vi "RawToRH.vi"(2 "Data":u8[](array[numeric]), 5 "error in (no error)":errorcluster) -> (16 "RH":dbl, 19 "error out":errorcluster)   [LabVIEW 2019, in "SHT21.lvclass"]
uses:
  SHT21.lvclass
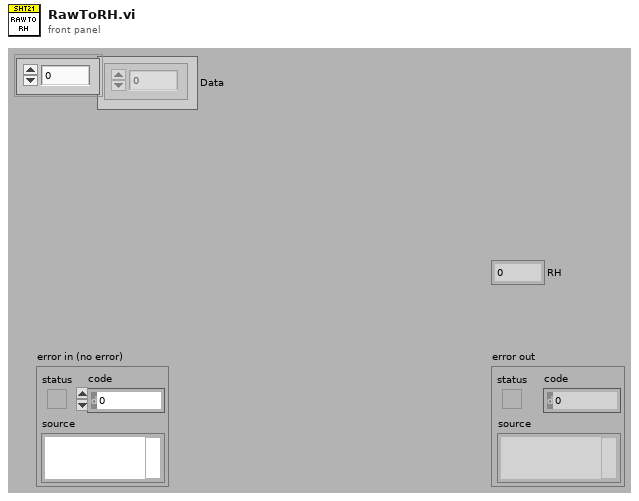
[diagram p1: front panel]
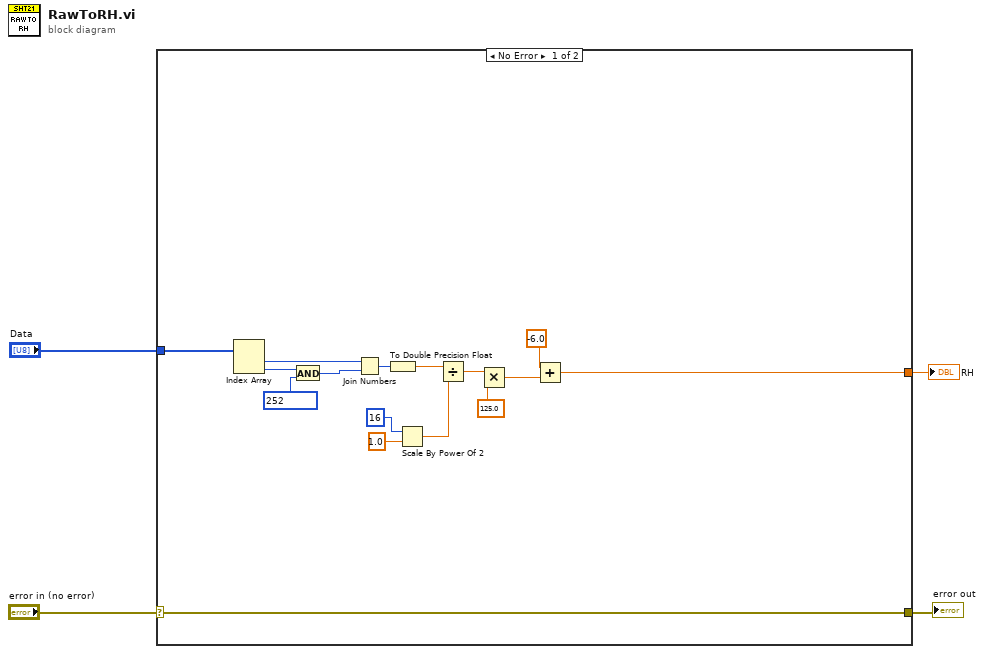
[diagram p0: block diagram]
diagram:
  n1 = case shown="No Error" "error in (no error)" {
    selector: "error in (no error)" -> [w20 w21]
    tunnel: [w20 w21] -> w3
    tunnel: "Data" -> [w5 _]
    tunnel: [w6 _] -> w1
    frame No Error {
      n2 = Index Array(array=w5) -> (element #1=w16:u8, element #2=w19:u8)  [unwired: 2 in]
      n3 = And(x=w19, y=u8 252) -> (x .and. y?=w17:u8)
      n4 = Join Numbers(hi=w16, lo=w17) -> ((hi.lo)=w15:u16)
      n5 = To Double Precision Float(number=w15) -> (double precision float=w14:dbl)
      n6 = Scale By Power Of 2(n=i16 16, x=1.0) -> (x*2^n=w11:dbl)
      n7 = Divide(x=w14, y=w11) -> (x/y=w10:dbl)
      n8 = Multiply(x=w10, y=125.0) -> (x*y=w8:dbl)
      n9 = Add(x=-6.0, y=w8) -> (x+y=w6:dbl)
    }
    frame Error {
    }
  }
  "error out" <- w3
  "RH" <- w1
